vi "Second Testbench.vi"   [LabVIEW 2015]
uses:
  Model Messages/Add VI from File Msg/Add VI from File Msg.lvclass
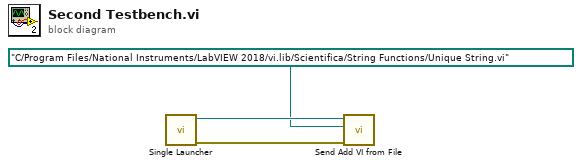
[diagram p0: block diagram]
diagram:
  n1 = call "Single Launcher.vi"() -> ("error out"=w2:errorcluster, "Documentation Tool Model"=w3:refnum<class "Message Enqueuer.lvclass">)  [unwired: 10 in]
  n2 = call "Send Add VI from File.vi"("error in (no error)"=w2, "VI Path"=path "C:/Program Files/National Instruments/LabVIEW 2018/vi.lib/Scientifica/String Functions/Unique String.vi", "Message Enqueuer"=w3) -> ()  [unwired: 7 in, 2 out]
